vi "Check_End_Position_PN.vi"(4 "Model       Roll      Pitch       Yaw (deg)":dbl[](array[numeric]) format="%#.2f", 7 "Traverse Name":string, 10 "New Position":dbl[](array[numeric])=[0.0, 0.0, 0.0] format="%.2f", 11 "Current position":dbl[](array[numeric])=[0.0, 0.0, 0.0] format="%.2f") -> (0 "Error Comments":string)   [LabVIEW 2014]
uses:
  <vilib>/Utility/miscctls.llb/LV3DPointTypeDef.ctl
  Globals/Constants_global.vi
panel:
  # "X                Y                   Z"
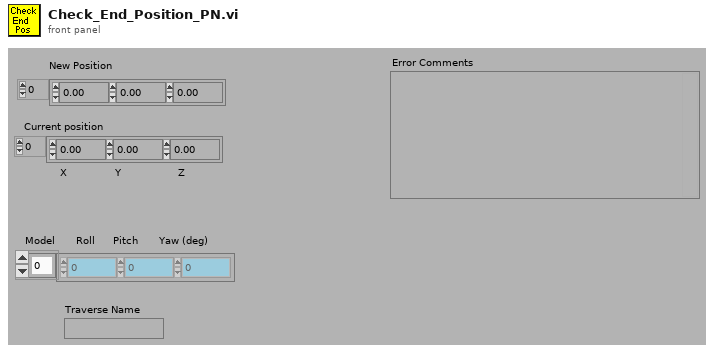
[diagram p1: front panel]
types:
  T1 = typedef "LV3DPointTypeDef.ctl" = cluster{"X":sgl, "Y":sgl, "Z":sgl}
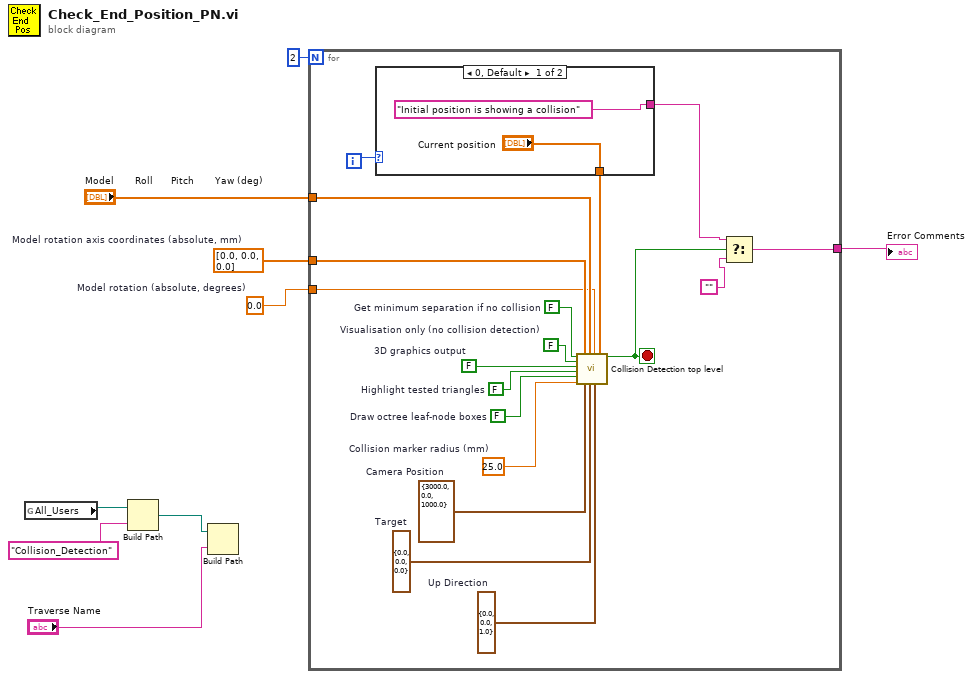
[diagram p0: block diagram]
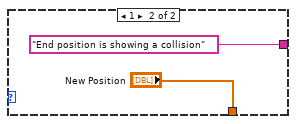
[diagram p2: hidden frame]
diagram:
  w5 = sgl 0.0  # Model rotation (absolute, degrees)
  w6 = sgl[] [0.0, 0.0, 0.0]  # Model rotation axis coordinates (absolute, mm)
  n1 = global read "Constants_global.vi" "All_Users"() -> (w4:path)
  n2 = Build Path(base path=w4, name or relative path="Collision_Detection") -> (appended path=w2:path)
  n3 = Build Path(base path=w2, name or relative path="Traverse Name") -> ()  [unwired: 1 out]
  n4 = for {
    N: 2 -> [_]
    tunnel: "Model       Roll      Pitch       Yaw (deg)" -> [w26]
    tunnel: [w16] -> w7
    tunnel: w6 -> [w11]
    tunnel: w5 -> [w10]
    i -> [w27]
    stop <- w19 stop-if-true
    w12 = T1 {"X"=0.0, "Y"=0.0, "Z"=1.0}  # Up Direction
    w13 = T1 {"X"=0.0, "Y"=0.0, "Z"=0.0}  # Target
    w14 = T1 {"X"=3000.0, "Y"=0.0, "Z"=1000.0}  # Camera Position
    w15 = sgl 25.0  # Collision marker radius (mm)
    w20 = FALSE  # Draw octree leaf-node boxes
    w21 = FALSE  # Highlight tested triangles
    w22 = FALSE  # 3D graphics output
    w23 = FALSE  # Visualisation only (no collision detection)
    w24 = FALSE  # Get minimum separation if no collision
    n5 = case shown="0, Default" w27 {
      tunnel: ["Current position" "New Position"] -> w25
      tunnel: ["Initial position is showing a collision" "End position is showing a collision"] -> w18
      frame 0, Default {
      }
      frame 1 {
      }
    }
    n6 = call "Collision Detection top level.vi"("Get minimum separation if no collision"=w24, "Visualisation only (no collision detection)"=w23, "3D graphics output"=w22, "Highlight tested triangles"=w21, "Draw octree leaf-node boxes"=w20, "Collision marker radius (mm)"=w15, "Model rotation axis coordinates (absolute, mm)"=w11, "Camera Position"=w14, "Model rotation axis (unit vector)"=w26, "Target"=w13, "Model rotation (absolute, degrees)"=w10, "Up Direction"=w12, "Traverse position (absolute, mm)"=w25) -> ("Collision"=w19:bool)  [unwired: 2 in, 4 out]
    n7 = Select(t=w18, s=w19, f="") -> (s? t:f=w16:string)
  }
  "Error Comments" <- w7
